vi "Drive to Distance ramp.vi"(8 "in":bool, 10 "Distance":dbl) -> (0 "next":bool)   [LabVIEW 2017]
uses:
  <vilib>/Rock Robotics/WPI/RobotDrive/WPI_RobotDriveArcadeDrive_Standard(NoSaturation).vi
  Robot Global Data.vi
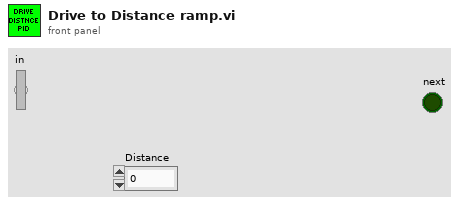
[diagram p1: front panel]
types:
  T1 = typedef "WPI_EncoderDevRef.ctl" = cluster{"DevStatus":errorcluster, "EncoderIndex":T2, "CounterIndex":T3, "DistancePerCount":dbl, "Decoding Type":T4}
  T2 = typedef "FPGA_EncoderIdx.ctl" = enum8{"Enc 0", "Enc 1", "Enc 2", "Enc 3", "Enc 4", "Enc 5", "Enc 6", "Enc 7", "Invalid"}
  T3 = typedef "FPGA_CounterCtrSystemIndex.ctl" = enum8{"Ctr 0", "Ctr 1", "Ctr 2", "Ctr 3", "Ctr 4", "Ctr 5", "Ctr 6", "Ctr 7", "Invalid"}
  T4 = typedef "WPI_EncoderType.ctl" = enum16{"1x", "2x", "4x"}
  T5 = typedef "WPI_RobotDriveDevRef.ctl" = cluster{"DevStatus":errorcluster, "Motors[]":T6[], "Square Inputs":bool, "Max Output":dbl}
  T6 = typedef "WPI_MotorControlDeviceRef.ctl" = cluster{"DeviceStatus":errorcluster, "Type":T7, "PWM":cluster{"PWM Channel":T8, "DeadBand":T9}, "CAN":cluster{"Device Number":u8, "SetOutput VI Ref":variant, "GetOutput VI Ref":variant, "Enable VI Ref":variant, "Disable VI Ref":variant, "Data":variant}, "Invert":bool, "DIO PWM":cluster{"PWM \"Enable\" Channel":T8, "DIOChannel":T10, "PWM Rate":dbl}}
  T7 = typedef "WPI_MotorControlType.ctl" = enum16{"PWM", "CAN", "DIO PWM"}
  T8 = typedef "FPGA_DIOPWMChannel.ctl" = enum8{"PWM 0", "PWM 1", "PWM 2", "PWM 3", "PWM 4", "PWM 5", "PWM 6", "PWM 7", "PWM 8", "PWM 9", "PWM MXP 0", "PWM MXP 1", "PWM MXP 2", "PWM MXP 3", "PWM MXP 4", "PWM MXP 5", "PWM MXP 6", "PWM MXP 7", "PWM MXP 8", "PWM MXP 9", "Invalid"}
  T9 = typedef "WPI_PWMDeadband.ctl" = cluster{"Name":string, "maxPositivePwm":i32, "minPositivePwm":i32, "centerPwm":i32, "maxNegativePwm":i32, "minNegativePwm":i32, "angularRange":u16}
  T10 = typedef "FPGA_DIOChannel.ctl" = enum8{"DIO 0", "DIO 1", "DIO 2", "DIO 3", "DIO 4", "DIO 5", "DIO 6", "DIO 7", "DIO 8", "DIO 9", "DIO MXP 0", "DIO MXP 1", "DIO MXP 2", "DIO MXP 3", "DIO MXP 4", "DIO MXP 5", "DIO MXP 6", "DIO MXP 7", "DIO MXP 8", "DIO MXP 9", "DIO MXP 10", "DIO MXP 11", "DIO MXP 12", "DIO MXP 13", "DIO MXP 14", "DIO MXP 15", "SPI Port CS1", "SPI Port CS2", "SPI Port CS3", "SPI Port MISO", "SPI Port MOSI", "Invalid"}
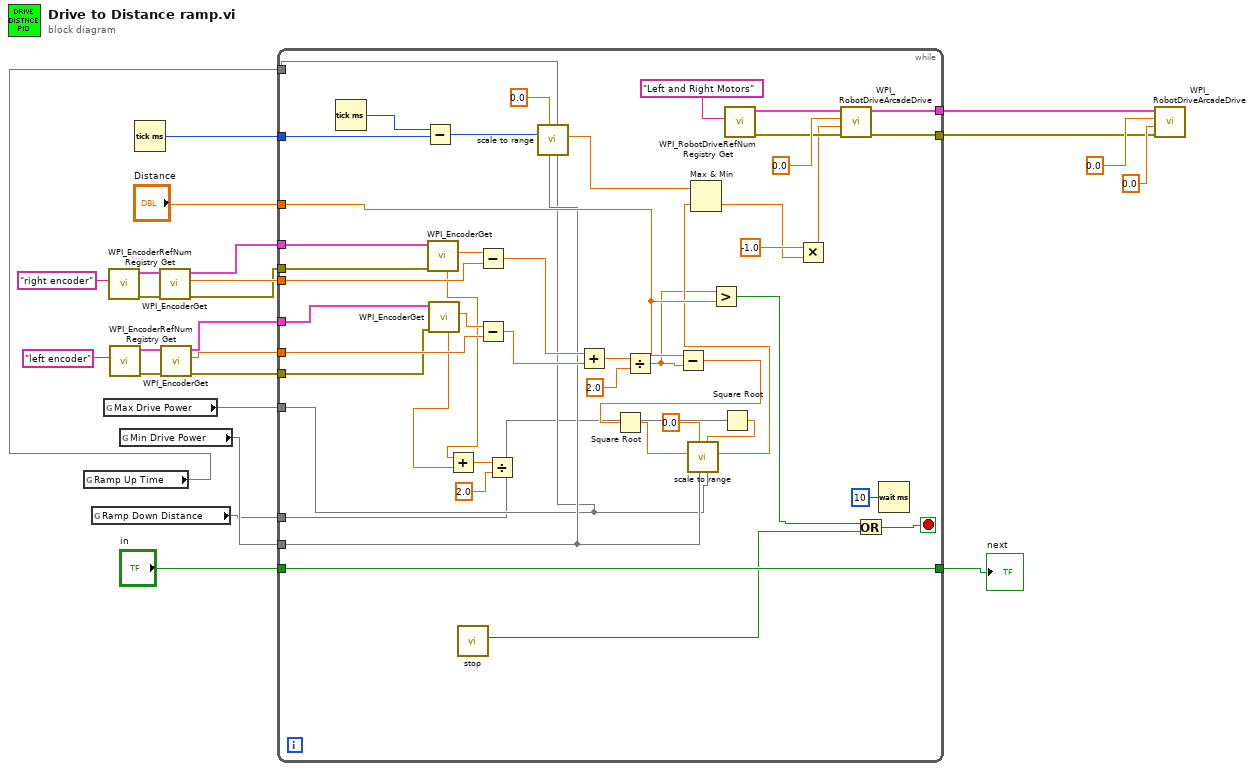
[diagram p0: block diagram]
diagram:
  n1 = global read "Robot Global Data.vi" "Ramp Up Time"() -> (w2)
  n2 = global read "Robot Global Data.vi" "Ramp Down Distance"() -> (w1)
  n3 = global read "Robot Global Data.vi" "Max Drive Power"() -> (w3)
  n4 = call <vilib>:"WPI_EncoderRefNum Registry Get.vi"("refnum name"="right encoder") -> ("error out"=w24:errorcluster, "EncoderDevRef"=w23:T1)  [unwired: 9 in]
  n5 = call <vilib>:"WPI_EncoderRefNum Registry Get.vi"("refnum name"="left encoder") -> ("error out"=w21:errorcluster, "EncoderDevRef"=w20:T1)  [unwired: 9 in]
  n6 = global read "Robot Global Data.vi" "Min Drive Power"() -> (w4)
  n7 = Tick Count (ms)() -> (millisecond timer value=w7:u32)
  n8 = call <vilib>:"WPI_EncoderGet.vi"("error in (no error)"=w24, "EncoderDevRef"=w23) -> ("error out"=w11:errorcluster, "Distance"=w18:dbl, "EncoderDevRef"=w12:T1)  [unwired: 4 in, 3 out]
  n9 = call <vilib>:"WPI_EncoderGet.vi"("error in (no error)"=w21, "EncoderDevRef"=w20) -> ("error out"=w10:errorcluster, "Distance"=w17:dbl, "EncoderDevRef"=w9:T1)  [unwired: 4 in, 3 out]
  n10 = while {
    tunnel: "Distance" -> [w48]
    tunnel: w18 -> [w63]
    tunnel: w17 -> [w64]
    tunnel: [w62] -> w14
    tunnel: [w61] -> w13
    tunnel: w12 -> [w60]
    tunnel: w11 -> [w59]
    tunnel: w10 -> [w58]
    tunnel: w9 -> [w57]
    tunnel: w7 -> [w42]
    tunnel: [w34] -> w6
    tunnel: "in" -> [w34]
    tunnel: w4 -> [w33]
    tunnel: w3 -> [w32]
    tunnel: w2 -> [w31]
    tunnel: w1 -> [w28]
    stop <- w26 stop-if-true
    n11 = Tick Count (ms)() -> (millisecond timer value=w41:u32)
    n12 = Subtract(x=w41, y=w42) -> (x-y=w35:u32)
    n13 = call <vilib>:"WPI_EncoderGet.vi"("error in (no error)"=w59, "EncoderDevRef"=w60) -> ("Distance"=w66:dbl, "Rate"=w53:dbl)  [unwired: 4 in, 4 out]
    n14 = call <vilib>:"WPI_EncoderGet.vi"("error in (no error)"=w58, "EncoderDevRef"=w57) -> ("Distance"=w65:dbl, "Rate"=w54:dbl)  [unwired: 4 in, 4 out]
    n15 = Add(x=w53, y=w54) -> (x+y=w56:dbl)
    n16 = call "stop.vi"() -> ("Boolean"=w27:bool)  [unwired: 11 in]
    n17 = Subtract(x=w66, y=w63) -> (x-y=w50:dbl)
    n18 = Subtract(x=w65, y=w64) -> (x-y=w49:dbl)
    n19 = Divide(x=w56, y=2.0) -> ()  [unwired: 1 out]
    n20 = call "scale to range.vi"("Max"=w32, "High"=w31, "Min"=w33, "Low"=0.0, "In Signal"=w35) -> ("Output signal"=w38:dbl)  [unwired: 6 in]
    n21 = Add(x=w50, y=w49) -> (x+y=w52:dbl)
    n22 = Divide(x=w52, y=2.0) -> (x/y=w36:dbl)
    n23 = Subtract(x=w48, y=w36) -> (x-y=w30:dbl)
    n24 = Square Root(x=w30) -> (sqrt(x)=w44:dbl)
    n25 = Greater?(x=w36, y=w48) -> (0:w25:bool)
    n26 = Square Root(x=w28) -> (sqrt(x)=w29:dbl)
    n27 = call "scale to range.vi"("Max"=w32, "High"=w29, "Min"=w33, "Low"=0.0, "In Signal"=w44) -> ("Output signal"=w39:dbl)  [unwired: 6 in]
    n28 = Max & Min(x=w38, y=w39) -> (min(x,y)=w37:dbl)  [unwired: 1 out]
    n29 = call <vilib>:"WPI_RobotDriveRefNum Registry Get.vi"("refnum name"="Left and Right Motors") -> ("error out"=w68:errorcluster, "RobotDriveDevRef"=w67:T5)  [unwired: 1 in, 8 out]
    n30 = Multiply(x=-1.0, y=w37) -> (x*y=w47:dbl)
    n31 = call-poly <vilib>:"WPI_RobotDriveArcadeDrive.vi"("error in (no error)"=w68, "Y axis value"=w47, "X axis value"=0.0, "RobotDriveDevRef"=w67) -> ("error out"=w62:errorcluster, "RobotDriveDevRef"=w61:T5)  [unwired: 6 out]
    n32 = Or(x=w25, y=w27) -> (x .or. y?=w26:bool)
    n33 = Wait (ms)(milliseconds to wait=u32 10) -> ()  [unwired: 1 out]
  }
  "next" <- w6
  n34 = call-poly <vilib>:"WPI_RobotDriveArcadeDrive.vi"("error in (no error)"=w14, "Y axis value"=0.0 ("X axis value"), "X axis value"=0.0, "RobotDriveDevRef"=w13) -> ()  [unwired: 8 out]
